vi "SR430_query_error_status_byte.vi"(0 "address":T2, 5 "error in (no error)":errorcluster) -> (14 "address out":T2, 16 "instrumentErrorStatusByte":T1, 19 "error out":errorcluster)   [LabVIEW 2009, in "SR430Driver.lvlib"]
doc: "Queries the error status byte\n\nCopyright (C)\nGesellschaft für Schwerionenforschung, GSI\nPlanckstr. 1\n64291 Darmstadt\nGermany\n\nContact: D.Beck@gsi.de \n\nThis program is free software; you can redistribute it and/or modify it under the terms of the \nGNU General Public License as published by the Free Software Foundation; either version 2 of the license, or (at your option) any later version.\n\nThis program is distributed in the hope that it will be useful, but WITHOUT ANY WARRANTY; without even the implied warranty of MERCHANTABILITY or FITNESS FOR A PARTICULAR PURPOSE. See the GNU General License for more details (http://www.gnu.org).\n\nGesellschaft für Schwerionenforschung, GSI\nPlanckstr. 1, 64291 Darmstadt, Germany\nFor all questions and ideas contact: M.Richter@gsi.de, K.Poppensieker, H.Brand@gsi.de or D.Beck@gsi.de.\nLast update: 11-APR-2002"
uses:
  SR430Driver.lvlib
  SR430_VISA Control.ctl
  SR430_errorStatusByte.ctl
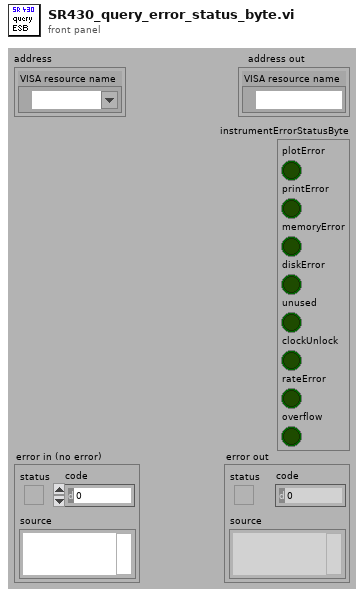
[diagram p1: front panel]
types:
  T1 = typedef "SR430Driver.lvlib/SR430_errorStatusByte.ctl" = cluster{"plotError":bool, "printError":bool, "memoryError":bool, "diskError":bool, "unused":bool, "clockUnlock":bool, "rateError":bool, "overflow":bool}
  T2 = typedef "SR430Driver.lvlib/SR430_VISA Control.ctl" = cluster{"VISA resource name":refnum<visa-resource-name>}
  T3 = cluster{"Boolean array[0]":bool, "Boolean array[1]":bool, "Boolean array[2]":bool, "Boolean array[3]":bool, "Boolean array[4]":bool, "Boolean array[5]":bool, "Boolean array[6]":bool, "Boolean array[7]":bool}
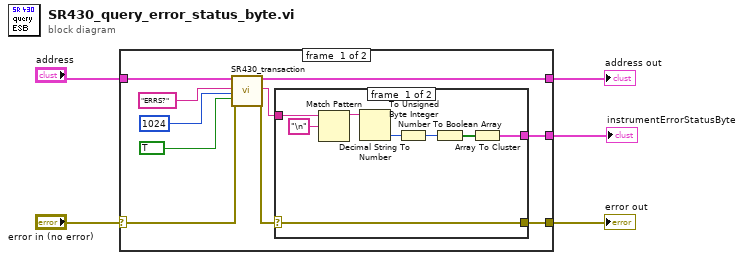
[diagram p0: block diagram]
diagram:
  n1 = case shown="No Error" "error in (no error)" {
    selector: "error in (no error)" -> [w13 w25]
    tunnel: "address" -> [w15 w26]
    tunnel: [w14 w26] -> w2
    tunnel: [w8 w25] -> w4
    tunnel: [w6 _] -> w1
    frame #0 {
      n2 = call "SR430_transaction.vi"("SR430 VISA Cluster"=w15, "SR430 Command String"="ERRS?", "Bytes to read (1024)"=u32 1024, "Read (FALSE)"=TRUE, "error in (no error)"=w13) -> ("dup SR430 VISA Cluster"=w14:T2, "SR430 Response"=w7:string, "error out"=w9:errorcluster)  [unwired: 11 in, 1 out]
      n3 = case shown="No Error" w9 {
        selector: w9 -> [w23 w24]
        tunnel: [w23 w24] -> w8
        tunnel: w7 -> [w20 _]
        tunnel: [w16 _] -> w6
        frame #0 {
          n4 = Match Pattern(string=w20, regular expression="\n") -> (before substring=w22:string)  [unwired: 1 in, 3 out]
          n5 = Decimal String To Number(string=w22) -> (number=w19:i32)  [unwired: 2 in, 1 out]
          n6 = To Unsigned Byte Integer(number=w19) -> (unsigned 8bit integer=w18:u8)
          n7 = Number To Boolean Array(number=w18) -> (Boolean array=w17:bool[])
          n8 = Array To Cluster(array=w17) -> (cluster=w16:T3)
        }
        frame #1 {
        }
      }
    }
    frame #1 {
    }
  }
  "error out" <- w4
  "address out" <- w2
  "instrumentErrorStatusByte" <- w1
